vi "Stoermeldungen Aussortieren fuer Anzeige.vi"(9 "Störmeldung":T1, 11 "Anzeige Array":T1[](array[typedef])) -> (3 "Anzeige Array":T1[](array[typedef]))   [LabVIEW 2020, in "Stoerungen.lvlib"]
uses:
  Stoerungen.lvlib
  Stoermeldung.ctl
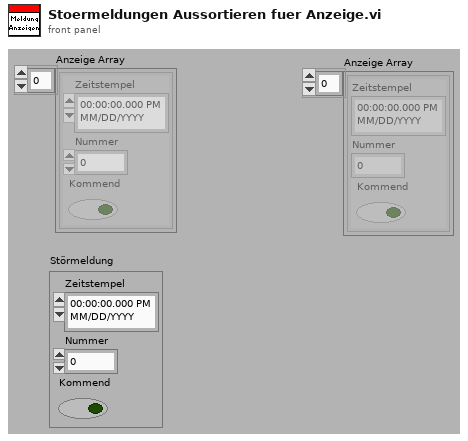
[diagram p1: front panel]
types:
  T1 = typedef "Stoerungen.lvlib/Stoermeldung.ctl" = cluster{"Zeitstempel":timestamp, "Nummer":i32, "Kommend":bool}
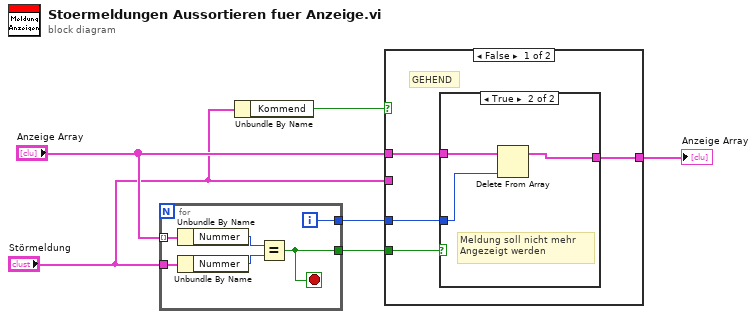
[diagram p0: block diagram]
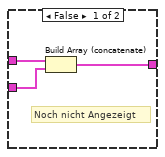
[diagram p4: hidden frame]
diagram:
  n1 = for {
    tunnel: "Anzeige Array" -> [w12] mode=indexing
    tunnel: "Störmeldung" -> [w11]
    tunnel: [w8] -> w5
    tunnel: [w7] -> w1
    i -> [w7]
    stop <- w8 stop-if-true
    n2 = Unbundle By Name(w12) -> ("Nummer"=w10:i32)
    n3 = Unbundle By Name(w11) -> ("Nummer"=w9:i32)
    n4 = Equal?(x=w10, y=w9) -> (x = y?=w8:bool)
  }
  n5 = Unbundle By Name("Störmeldung") -> ("Kommend"=w2:bool)
  n6 = case shown="False" w2 {
    tunnel: [w13 w24] -> w6
    tunnel: w5 -> [w16 w23]
    tunnel: "Anzeige Array" -> [w14 w22]
    tunnel: "Störmeldung" -> [_ w21]
    tunnel: w1 -> [w15 _]
    frame False {
      # "GEHEND"
      n7 = case shown="True" w16 {
        tunnel: w14 -> [w17 w20]
        tunnel: [w17 w18] -> w13
        tunnel: w15 -> [_ w19]
        frame False {
          # "Meldung nicht gefunden"
        }
        frame True {
          # "Meldung soll nicht mehr \nAngezeigt werden"
          n8 = Delete From Array(array=w20, index=w19) -> (array with subset deleted=w18:T1[])  [unwired: 1 in, 1 out]
        }
      }
    }
    frame True {
      # "KOMMEND"
      n9 = case shown="True" w23 {
        tunnel: w22 -> [w27 w28]
        tunnel: [w25 w28] -> w24
        tunnel: w21 -> [w26 _]
        frame False {
          # "Noch nicht Angezeigt"
          n10 = Build Array (concatenate)(w27, w26) -> (w25:T1[])
        }
        frame True {
          # "Wird schon Angezeigt"
        }
      }
    }
  }
  "Anzeige Array" <- w6
